vi "GetImage.vi"(0 "XRef":T4, 1 "State In":T3) -> (14 "Image":T2, 15 "Fatal Error Out":T1)   [LabVIEW 2015, in "Get Object Parameters.xnode"]
uses:
  Get Object Parameters.xnode
  <vilib>/XNodeSupport/XNodeXNodeRef.ctl
  State.ctl
  <vilib>/XNodeSupport/XNodeImage.ctl
  <vilib>/XNodeSupport/XNodeErrorCluster.ctl
  dimensions.vi
  <vilib>/XNodeSupport/NI_XNodeSupport.lvlib
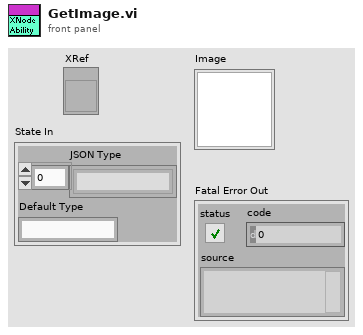
[diagram p1: front panel]
types:
  T1 = typedef "NI_XNodeSupport.lvlib/XNodeErrorCluster.ctl" = errorcluster
  T2 = typedef "NI_XNodeSupport.lvlib/XNodeImage.ctl" = picture
  T3 = typedef "Get Object Parameters.xnode/State.ctl" = cluster{"JSON Type":string[], "Default Type":string}
  T4 = typedef "NI_XNodeSupport.lvlib/XNodeXNodeRef.ctl" = refnum<vi>
  T5 = typedef "imagedata.ctl" = cluster{"image type":i32, "image depth":i32, "image":u8[], "mask":u8[], "colors":u32[], "Rectangle":cluster{"left":i16, "top":i16, "right":i16, "bottom":i16}}
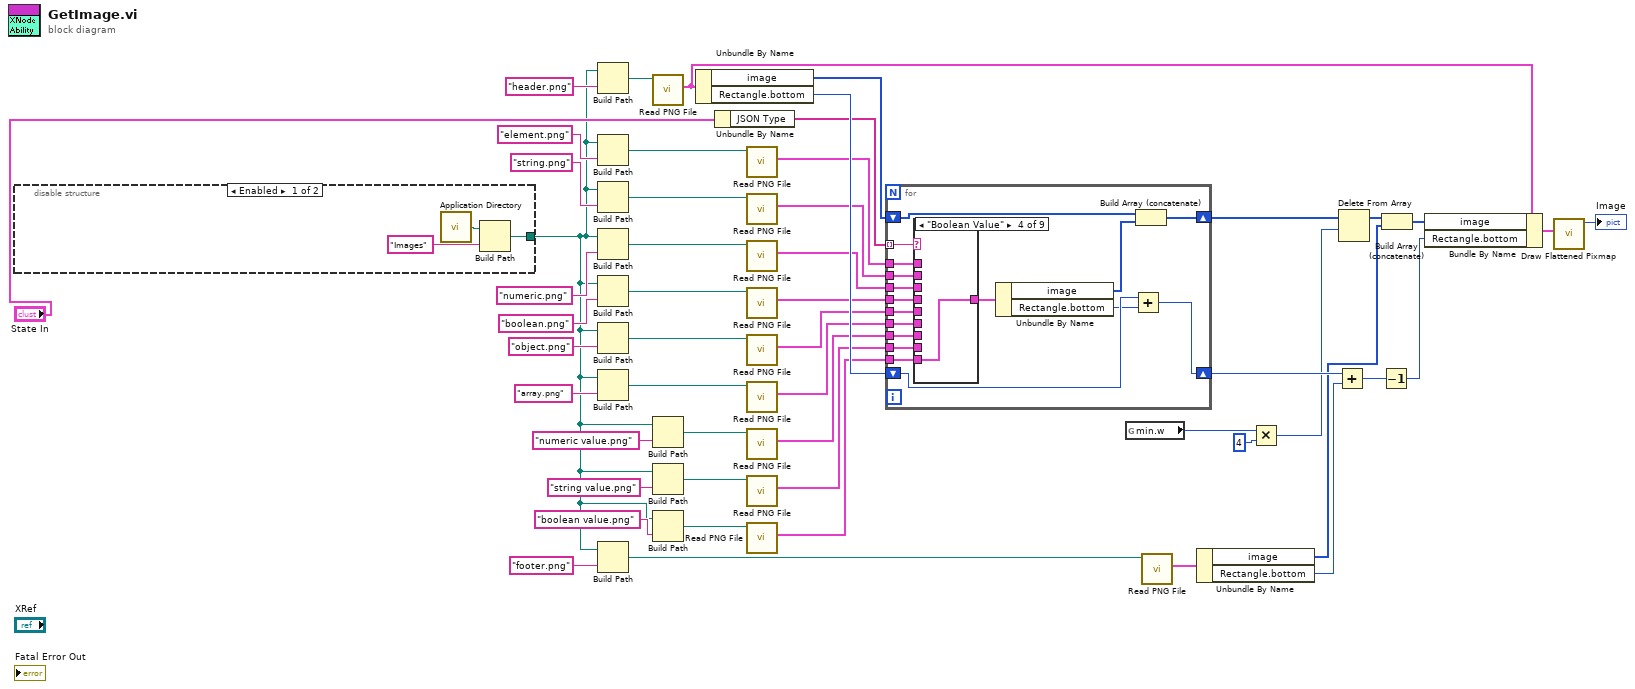
[diagram p0: block diagram]
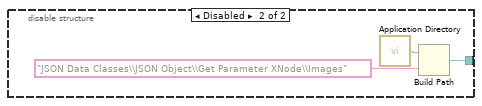
[diagram p10: hidden frame]
diagram:
  n1 = disable-structure shown="Enabled" {
    disable-tunnel: [w53 w56] -> w1
    frame Enabled {
      n2 = call <vilib>:"Application Directory.vi"() -> ("Application Directory"=w52:path)
      n3 = Build Path(base path=w52, name or relative path="Images") -> (appended path=w53:path)
    }
    frame Disabled {
      n4 = call <vilib>:"Application Directory.vi"() -> ("Application Directory"=w55:path)
      n5 = Build Path(base path=w55, name or relative path="JSON Data Classes\\JSON Object\\Get Parameter XNode\\Images") -> (appended path=w56:path)
    }
  }
  n6 = Build Path(base path=w1, name or relative path="header.png") -> (appended path=w47:path)
  n7 = Build Path(base path=w1, name or relative path="element.png") -> (appended path=w46:path)
  n8 = Build Path(base path=w1, name or relative path="string.png") -> (appended path=w33:path)
  n9 = Build Path(base path=w1, name or relative path="numeric.png") -> (appended path=w26:path)
  n10 = Build Path(base path=w1, name or relative path="boolean.png") -> (appended path=w24:path)
  n11 = Build Path(base path=w1, name or relative path="object.png") -> (appended path=w22:path)
  n12 = Build Path(base path=w1, name or relative path="array.png") -> (appended path=w23:path)
  n13 = Build Path(base path=w1, name or relative path="footer.png") -> (appended path=w45:path)
  n14 = call <vilib>:"Read PNG File.vi"("path to PNG file"=w47) -> ("image data"=w51:T5)  [unwired: 8 in, 2 out]
  n15 = Build Path(base path=w1, name or relative path="numeric value.png") -> (appended path=w3:path)
  n16 = Build Path(base path=w1, name or relative path="string value.png") -> (appended path=w6:path)
  n17 = Build Path(base path=w1, name or relative path="boolean value.png") -> (appended path=w7:path)
  n18 = Unbundle By Name(w51) -> ("image"=w43:u8[], "Rectangle.bottom"=w41:i16)
  n19 = Unbundle By Name("State In") -> ("JSON Type"=w35:string[])
  n20 = call <vilib>:"Read PNG File.vi"("path to PNG file"=w46) -> ("image data"=w31:T5)  [unwired: 8 in, 2 out]
  n21 = call <vilib>:"Read PNG File.vi"("path to PNG file"=w33) -> ("image data"=w32:T5)  [unwired: 8 in, 2 out]
  n22 = call <vilib>:"Read PNG File.vi"("path to PNG file"=w26) -> ("image data"=w25:T5)  [unwired: 8 in, 2 out]
  n23 = call <vilib>:"Read PNG File.vi"("path to PNG file"=w24) -> ("image data"=w21:T5)  [unwired: 8 in, 2 out]
  n24 = call <vilib>:"Read PNG File.vi"("path to PNG file"=w22) -> ("image data"=w19:T5)  [unwired: 8 in, 2 out]
  n25 = call <vilib>:"Read PNG File.vi"("path to PNG file"=w23) -> ("image data"=w20:T5)  [unwired: 8 in, 2 out]
  n26 = call <vilib>:"Read PNG File.vi"("path to PNG file"=w3) -> ("image data"=w4:T5)  [unwired: 8 in, 2 out]
  n27 = call <vilib>:"Read PNG File.vi"("path to PNG file"=w6) -> ("image data"=w5:T5)  [unwired: 8 in, 2 out]
  n28 = call <vilib>:"Read PNG File.vi"("path to PNG file"=w7) -> ("image data"=w2:T5)  [unwired: 8 in, 2 out]
  n29 = for {
    shift-right: [w71] -> w17
    shift-left: w43 -> [w74]
    shift-right: [w72] -> w40
    shift-left: w41 -> [w73]
    tunnel: w35 -> [w70] mode=indexing
    tunnel: w32 -> [w69]
    tunnel: w31 -> [w66]
    tunnel: w25 -> [w65]
    tunnel: w21 -> [w64]
    tunnel: w20 -> [w63]
    tunnel: w19 -> [w62]
    tunnel: w5 -> [w60]
    tunnel: w4 -> [w59]
    tunnel: w2 -> [w58]
    n30 = case shown="\"Boolean Value\"" w70 {
      tunnel: w69 -> [_ _ _ _ w79 _ _ _ _]
      tunnel: [w75 w76 w77 w78 w79 w80 w81 w82 w83] -> w68
      tunnel: w66 -> [w75 _ _ _ _ _ _ _ _]
      tunnel: w65 -> [_ _ _ _ _ w80 _ _ _]
      tunnel: w64 -> [_ _ _ _ _ _ w81 _ _]
      tunnel: w63 -> [_ _ _ _ _ _ _ w82 _]
      tunnel: w62 -> [_ _ _ _ _ _ _ _ w83]
      tunnel: w60 -> [_ w76 _ _ _ _ _ _ _]
      tunnel: w59 -> [_ _ w77 _ _ _ _ _ _]
      tunnel: w58 -> [_ _ _ w78 _ _ _ _ _]
      frame "JSON", Default {
      }
      frame "String Value" {
      }
      frame "Numeric Value" {
      }
      frame "Boolean Value" {
      }
      frame "JSON String" {
      }
      frame "JSON Numeric" {
      }
      frame "JSON Boolean" {
      }
      frame "JSON Array" {
      }
      frame "JSON Object" {
      }
    }
    n31 = Unbundle By Name(w68) -> ("image"=w67:u8[], "Rectangle.bottom"=w61:i16)
    n32 = Add(x=w73, y=w61) -> (x+y=w72:i16)
    n33 = Build Array (concatenate)(w74, w67) -> (w71:u8[])
  }
  n34 = global read "dimensions.vi" "min.w"() -> (w13:i32)
  n35 = call <vilib>:"Read PNG File.vi"("path to PNG file"=w45) -> ("image data"=w50:T5)  [unwired: 8 in, 2 out]
  n36 = Unbundle By Name(w50) -> ("image"=w39:u8[], "Rectangle.bottom"=w38:i16)
  n37 = Multiply(x=w13, y=4) -> (x*y=w11:i32)
  n38 = Add(x=w40, y=w38) -> (x+y=w15:i16)
  n39 = Delete From Array(array=w17, length=w11) -> (array with subset deleted=w16:u8[])  [unwired: 1 in, 1 out]
  n40 = Decrement(x=w15) -> (x-1=w14:i16)
  n41 = Build Array (concatenate)(w16, w39) -> (w18:u8[])
  n42 = Bundle By Name(cluster=w51, "image"=w18, "Rectangle.bottom"=w14) -> (w42:T5)
  n43 = call <vilib>:"Draw Flattened Pixmap.vi"("image data"=w42) -> ("new picture"=→"Image":picture)  [unwired: 8 in]
